vi "Get Refnum.vi"(8 "error in (no error)":errorcluster, 11 "QObject in":refnum<class "QObject.lvclass">) -> (0 "error out":errorcluster, 2 "Refnum":u32, 3 "QObject out":refnum<class "QObject.lvclass">)   [LabVIEW 2013, in "Template.lvlib" / "QObject.lvclass"]
uses:
  QObject.lvclass
  QObject.lvclass/QObject.ctl
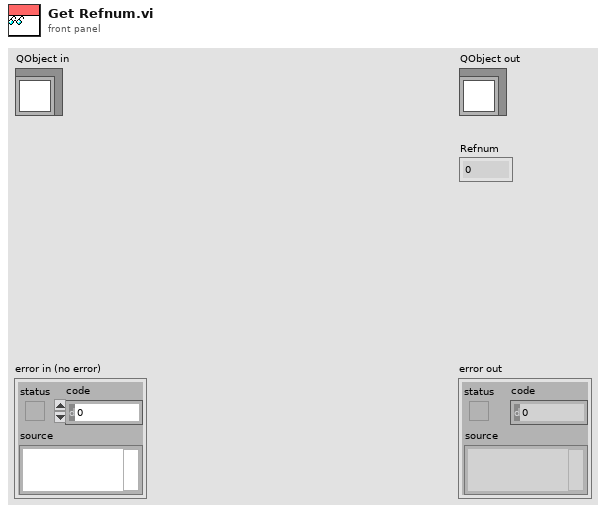
[diagram p1: front panel]
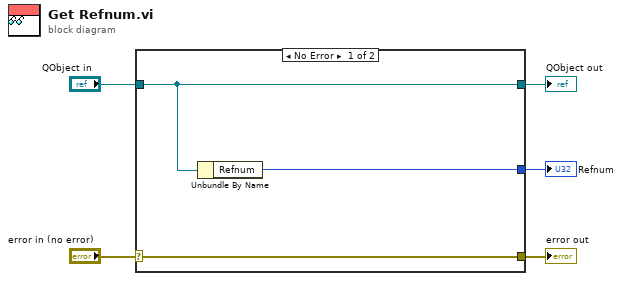
[diagram p0: block diagram]
diagram:
  n1 = case shown="No Error" "error in (no error)" {
    selector: "error in (no error)" -> [w8 w9]
    tunnel: [w8 w9] -> w4
    tunnel: [w7 w10] -> w2
    tunnel: "QObject in" -> [w7 w10]
    tunnel: [w6 _] -> w1
    frame No Error {
      n2 = Unbundle By Name(w7) -> ("Refnum"=w6:u32)
    }
    frame Error {
    }
  }
  "error out" <- w4
  "QObject out" <- w2
  "Refnum" <- w1
